vi "advanced-program.vi"() -> ()   [LabVIEW 2022 SP3]
uses:
  _driver/Basic driver/Communication/controls/comm_rate_enum.ctl
  _driver/_private/Control/Control Mode.ctl
  <vilib>/Instr/_visa.llb/VISA Find Search Mode.ctl
  _driver/_private/Control/Programmable Mode.ctl
  _driver/Chemyx_Syringe_Pump_driver.lvlib
panel:
  in  "error in (no error)":errorcluster
  out "error out":errorcluster
  in  "[x]":T1
  in  "Com Port":string(combo)
  in  "Volume (array)":dbl[](array[numeric])
  in  "Rate (array)":dbl[](array[numeric])
  in  "Diameter (mm)":dbl
  in  "Delay (min)":dbl[](array[numeric])
  in  "Pause":bool
  in  "Stop":bool
  in  "Start":bool
  in  "Baud rate":T2
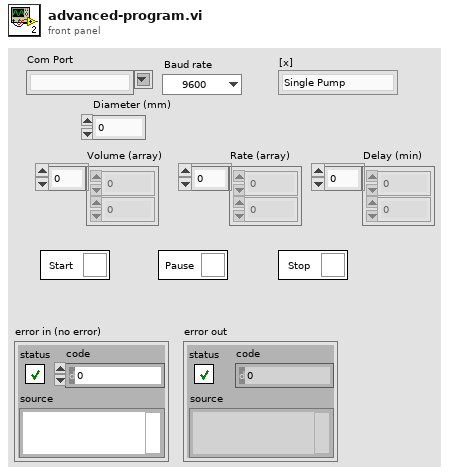
[diagram p1: front panel]
types:
  T1 = typedef "Chemyx_Syringe_Pump_driver.lvlib/Control Mode.ctl" = enum16{"Single Pump", "Pump Channel 1", "Pump Channel 2", "Cycle Mode"}
  T2 = typedef "Chemyx_Syringe_Pump_driver.lvlib/comm_rate_enum.ctl" = enum16{"9600", "38400"}
  T3 = typedef "VISA Find Search Mode.ctl" = u32
  T4 = typedef "Chemyx_Syringe_Pump_driver.lvlib/Programmable Mode.ctl" = enum16{"Blank", "Basic", "Programmable"}
  T5 = enum32{"invalid app kind", "Development System", "Run Time System", "Student Edition", "Embedded LabVIEW", "Evaluation", "Custom"}
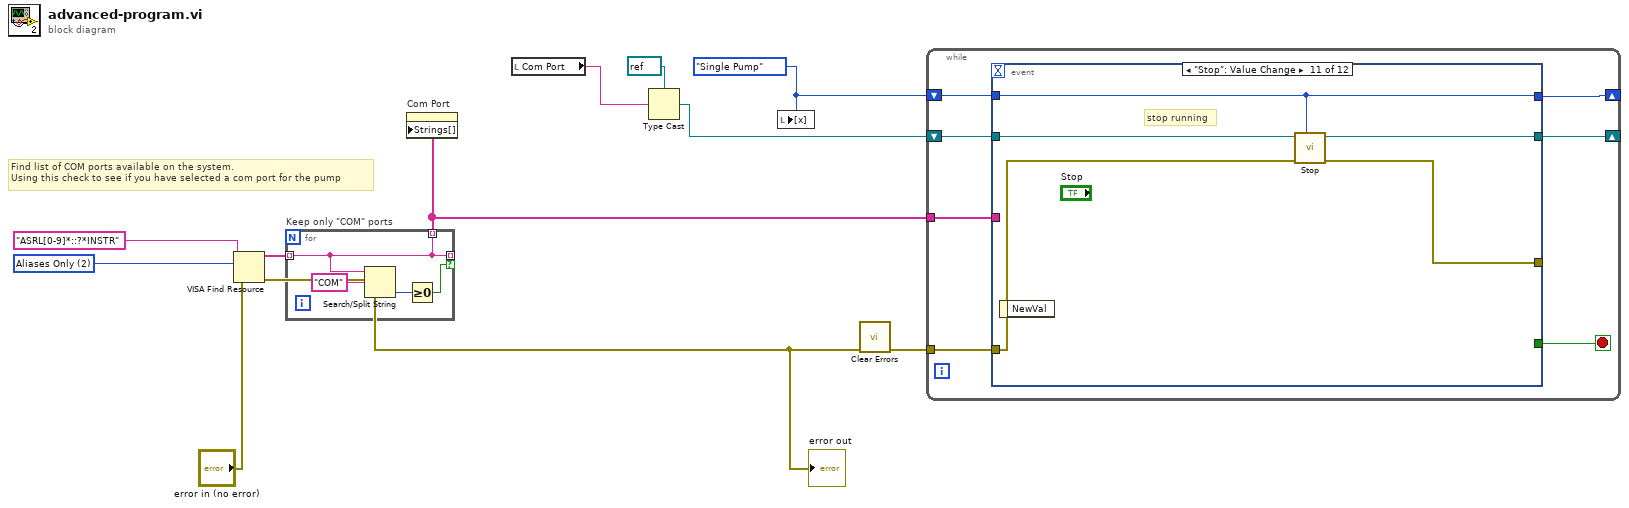
[diagram p0: block diagram]
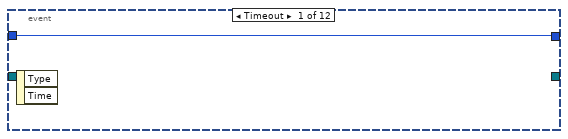
[diagram p2: hidden frame]
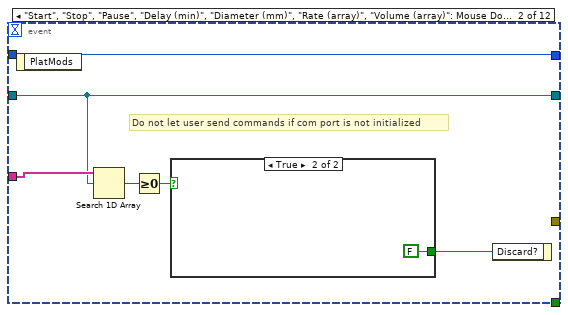
[diagram p3: hidden frame]
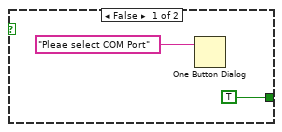
[diagram p4: hidden frame]
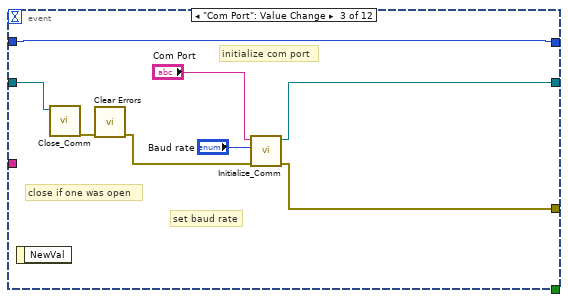
[diagram p5: hidden frame]
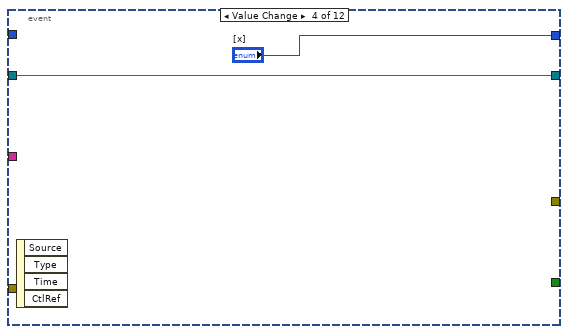
[diagram p6: hidden frame]
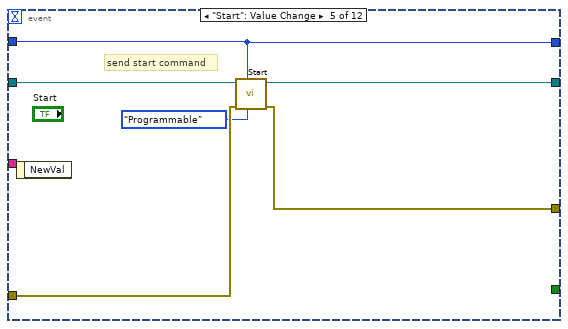
[diagram p7: hidden frame]
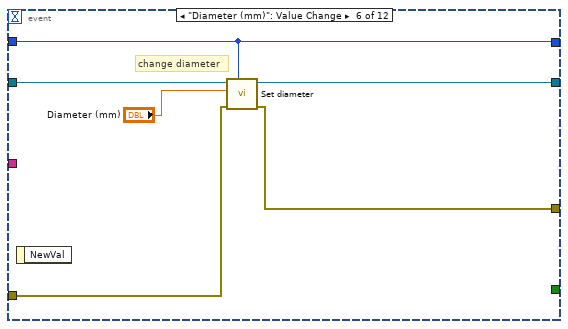
[diagram p8: hidden frame]
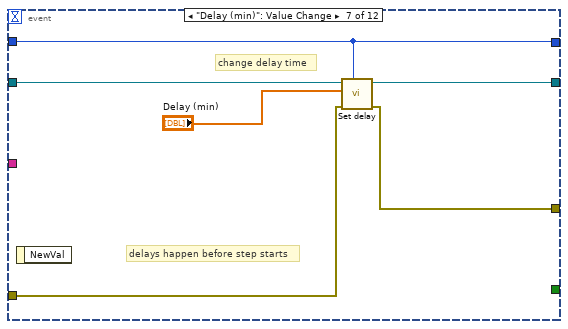
[diagram p9: hidden frame]
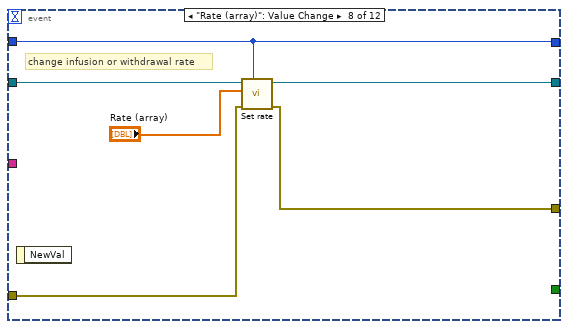
[diagram p10: hidden frame]
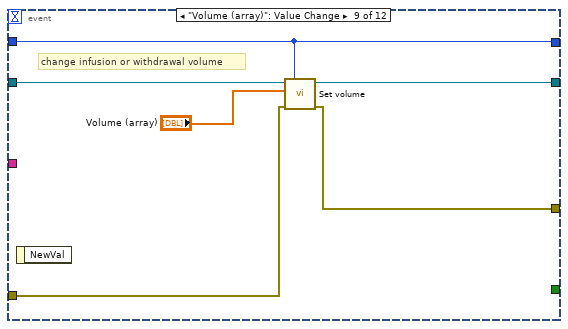
[diagram p11: hidden frame]
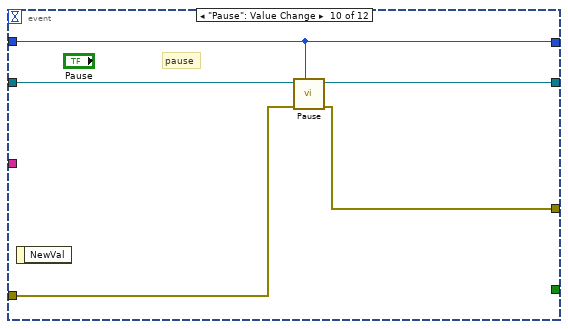
[diagram p12: hidden frame]
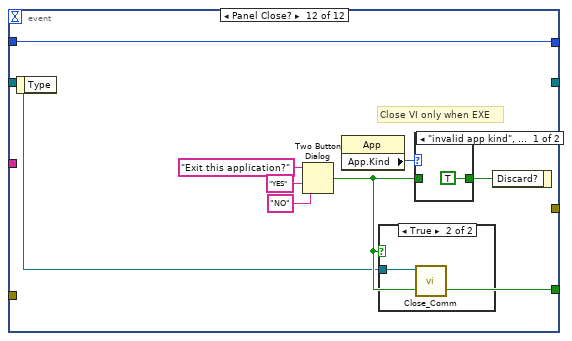
[diagram p13: hidden frame]
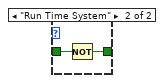
[diagram p15: hidden frame]
diagram:
  w4 = T3 2 items=["Canonical Names Only"=0, "Aliases Only"=2, "Include Matching Aliases"=3, "Include All Aliases"=4] ("Search Mode")
  w8 = Control_Mode."Single Pump" ("[x]")
  # "Find list of COM ports available on the system. \nUsing this check to see if you have selected a com port for the pump"
  n1 = VISA Find Resource(8:"error in (no error)", 10:w4, 11:"ASRL[0-9]*::?*INSTR" ("expression (\"?*\")")) -> (0:w1:errorcluster, 3:w6:string[])  [unwired: 1 out]
  "error out" <- w1
  n2 = for "Keep only \"COM\" ports" {
    tunnel: w6 -> [w12] mode=indexing
    tunnel: [w12] -> _ mode=indexing if=w13
    tunnel: [w12] -> w2 mode=indexing
    n3 = Search/Split String(string=w12, search string/char (-)="COM") -> (offset of match=w14:i32)  [unwired: 1 in, 2 out]
    n4 = Greater Or Equal To 0?(x=w14) -> (x >= 0?=w13:bool)
  }
  n5 = property on="Com Port" class="CmbBox"("Strings[]"=w2) -> ()  [unwired: 2 in, 2 out]
  n6 = local read "Com Port"() -> (w11:string)
  n7 = Type Cast(type=refnum<visa-resource-name> refnum ("Serial Port out"), x=w11) -> (*(type *) &x=w9:refnum<visa-resource-name>)
  n8 = local write "[x]"(w8) -> ()
  n9 = call <vilib>:"Clear Errors.vi"("error in (no error)"=w1) -> ("error out"=w7:errorcluster)  [unwired: 5 in, 1 out]
  n10 = while {
    shift-right: [w21] -> _
    shift-left: w9 -> [w20]
    tunnel: w2 -> [w19]
    tunnel: w7 -> [w18]
    shift-right: [w16] -> _
    shift-left: w8 -> [w17]
    stop <- w22 stop-if-true
    n11 = event shown="[10] \"Stop\": Value Change" {
      selector: _ -> [_ _ _ _ _ _ _ _ _ _ _ _]
      dyn-events: _ -> [_ _ _ _ _ _ _ _ _ _ _ _]
      timeout: _ -> [_ _ _ _ _ _ _ _ _ _ _ _]
      tunnel: [_ _ _ _ _ _ _ _ _ _ _ w85] -> w22
      tunnel: [_ w27 w39 w41 w48 w52 w58 w64 w70 w76 w81 _] -> w21
      tunnel: w20 -> [_ w27 w37 w41 w47 w53 w59 w65 w71 w77 w82 w84]
      tunnel: [_ _ w38 _ w46 w51 w57 w63 w69 w75 w80 _] -> _
      tunnel: w19 -> [_ w28 _ _ _ _ _ _ _ _ _ _]
      tunnel: w18 -> [_ _ _ _ w45 w50 w56 w62 w68 w74 w79 _]
      tunnel: w17 -> [w23 w24 w33 _ w44 w49 w55 w61 w67 w73 w78 w83]
      tunnel: [w23 w24 w33 "[x]" w44 w49 w55 w61 w67 w73 w78 w83] -> w16
      event Timeout {
        n12 = event-data() -> ()  [unwired: 1 in, 2 out]
      }
      event "Start", "Stop", "Pause", "Delay (min)", "Diameter (mm)", "Rate (array)", "Volume (array)": Mouse Down? {
        # "Do not let user send commands if com port is not initialized"
        n13 = event-data() -> ()  [unwired: 1 in, 1 out]
        n14 = Search 1D Array(1D array=w28, element=w27) -> (index of element=w29:i32)  [unwired: 1 in]
        n15 = Greater Or Equal To 0?(x=w29) -> (x >= 0?=w26:bool)
        n16 = case shown="True" w26 {
          tunnel: [TRUE FALSE] -> w25
          frame False {
            n17 = One Button Dialog(message="Pleae select COM Port") -> ()  [unwired: 1 in, 1 out]
          }
          frame True {
          }
        }
        n18 = event-data("Discard?"=w25) -> ()  [unwired: 1 in, 1 out]
      }
      event "Com Port": Value Change {
        # "set baud rate"
        # "close if one was open"
        # "initialize com port"
        n19 = event-data() -> ()  [unwired: 1 in, 1 out]
        n20 = call "Close_Comm.vi"("Serial Port in"=w37) -> ("error out"=w36:errorcluster)  [unwired: 10 in]
        n21 = call <vilib>:"Clear Errors.vi"("error in (no error)"=w36) -> ("error out"=w35:errorcluster)  [unwired: 5 in, 1 out]
        n22 = call "Initialize_Comm.vi"("error in (no error)"=w35, "Baud rate"="Baud rate", "Serial Port in"="Com Port") -> ("error out"=w38:errorcluster, "Serial Port out"=w39:refnum<visa-resource-name>)  [unwired: 7 in]
      }
      event Value Change {
        n23 = event-data() -> ()  [unwired: 1 in, 4 out]
      }
      event "Start": Value Change {
        # "send start command"
        n24 = event-data() -> ()  [unwired: 1 in, 1 out]
        n25 = call "Start.vi"("Mode"=Programmable_Mode."Programmable", "[x]"=w44, "error in (no error)"=w45, "Serial Port in"=w47) -> ("error out"=w46:errorcluster, "Serial Port out"=w48:refnum<visa-resource-name>)  [unwired: 6 in]
      }
      event "Diameter (mm)": Value Change {
        # "change diameter"
        n26 = event-data() -> ()  [unwired: 1 in, 1 out]
        n27 = call "Set diameter.vi"("[x]"=w49, "error in (no error)"=w50, "Diameter (mm)"="Diameter (mm)", "Serial Port in"=w53) -> ("error out"=w51:errorcluster, "Serial Port out"=w52:refnum<visa-resource-name>)  [unwired: 6 in]
      }
      event "Delay (min)": Value Change {
        # "delays happen before step starts"
        # "change delay time"
        n28 = event-data() -> ()  [unwired: 1 in, 1 out]
        n29 = call "Set delay.vi"("[x]"=w55, "error in (no error)"=w56, "Delay (min)"="Delay (min)", "Serial Port in"=w59) -> ("error out"=w57:errorcluster, "Serial Port out"=w58:refnum<visa-resource-name>)  [unwired: 6 in]
      }
      event "Rate (array)": Value Change {
        # "change infusion or withdrawal rate"
        n30 = event-data() -> ()  [unwired: 1 in, 1 out]
        n31 = call "Set rate.vi"("[x]"=w61, "error in (no error)"=w62, "Rate (array)"="Rate (array)", "Serial Port in"=w65) -> ("error out"=w63:errorcluster, "Serial Port out"=w64:refnum<visa-resource-name>)  [unwired: 6 in]
      }
      event "Volume (array)": Value Change {
        # "change infusion or withdrawal volume"
        n32 = event-data() -> ()  [unwired: 1 in, 1 out]
        n33 = call "Set volume.vi"("[x]"=w67, "error in (no error)"=w68, "Volume (array)"="Volume (array)", "Serial Port in"=w71) -> ("error out"=w69:errorcluster, "Serial Port out"=w70:refnum<visa-resource-name>)  [unwired: 6 in]
      }
      event "Pause": Value Change {
        # "pause"
        n34 = event-data() -> ()  [unwired: 1 in, 1 out]
        n35 = call "Pause.vi"("[x]"=w73, "error in (no error)"=w74, "Serial Port in"=w77) -> ("error out"=w75:errorcluster, "Serial Port out"=w76:refnum<visa-resource-name>)  [unwired: 7 in]
      }
      event "Stop": Value Change {
        # "stop running"
        n36 = event-data() -> ()  [unwired: 1 in, 1 out]
        n37 = call "Stop.vi"("[x]"=w78, "error in (no error)"=w79, "Serial Port in"=w82) -> ("error out"=w80:errorcluster, "Serial Port out"=w81:refnum<visa-resource-name>)  [unwired: 7 in]
      }
      event Panel Close? {
        # "Close VI only when EXE"
        n38 = event-data() -> ()  [unwired: 1 in, 1 out]
        n39 = Two Button Dialog(message="Exit this application?", 1:"NO" ("F button name (\"Cancel\")"), 2:"YES" ("T button name (\"OK\")")) -> (T button?=w85:bool)
        n40 = property class="App"() -> ("App.Kind"=w90:T5)  [unwired: 2 in, 2 out]
        n41 = case shown="True" w85 {
          tunnel: w84 -> [_ w91]
          frame False {
          }
          frame True {
            n42 = call "Close_Comm.vi"("Serial Port in"=w91) -> ()  [unwired: 10 in, 1 out]
          }
        }
        n43 = case shown="\"invalid app kind\", Default" w90 {
          tunnel: w85 -> [_ w94]
          tunnel: [TRUE ("Discard?") w93] -> w86
          frame "invalid app kind", Default {
          }
          frame "Run Time System" {
            n44 = Not(x=w94) -> (.not. x?=w93:bool)
          }
        }
        n45 = event-data("Discard?"=w86) -> ()  [unwired: 1 in, 1 out]
      }
    }
  }
